vi "captureBining.vi"(0 "Image in":T1, 1 "session in":refnum<k35>, 5 "imageBinned":T1, 7 "Cam ID":u32, 9 "Binning":u32, 11 "error in (no error)":errorcluster) -> (3 "session out":refnum<k35>, 4 "Image out":T1, 15 "error out":errorcluster)   [LabVIEW 2022 SP3]
uses:
  <vilib>/vision/Image Controls.llb/IMAQ Image.ctl
  <vilib>/vision/NI_Vision_Development_Module.lvlib
panel:
  in  "Image Size":cluster{"x":i32, "y":i32}
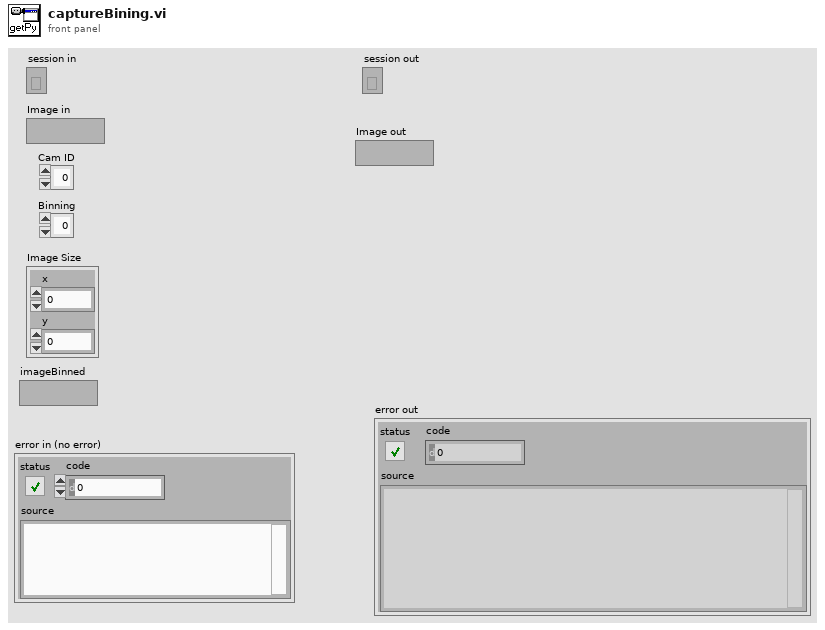
[diagram p1: front panel]
types:
  T1 = typedef "IMAQ Image.ctl" = refnum<image>
  T2 = cluster{"[0]":u32, "[1]":u32, "[2]":u32, "[3]":u32, "[4]":u32, "[5]":u32, "[6]":u32, "[7]":u32, "[8]":u32}
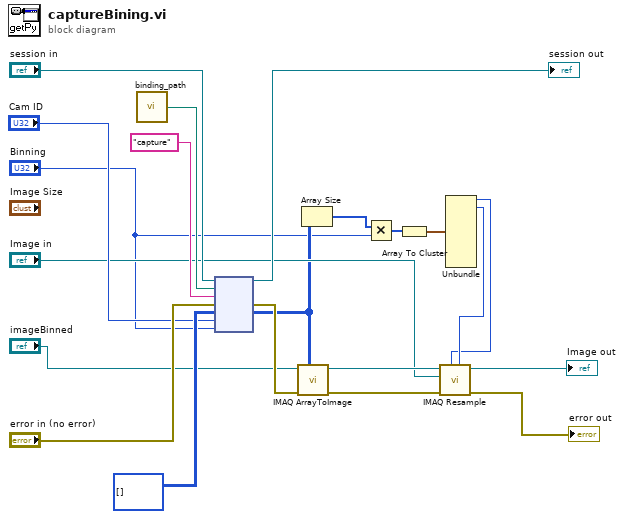
[diagram p0: block diagram]
diagram:
  n1 = call "binding_path.vi"() -> ("appended path"=w12:path)
  n2 = node("session in", w12, "capture" ("function name"), "error in (no error)", u16[][] [] ("image"), "Cam ID", "Binning") -> (→"session out":refnum<k35>, w15:errorcluster, w7:u16[][])  [unwired: 2 in, 2 out]
  n3 = call "IMAQ ArrayToImage"("Image Pixels (U16)"=w7, "error in (no error)"=w15, "Image"="imageBinned") -> ("error out"=w13:errorcluster, "Image Out"=w20:T1)  [unwired: 7 in]
  n4 = Array Size(array=w7) -> (size(s)=w6:i32[])
  n5 = Multiply(x=w6, y="Binning") -> (x*y=w4:u32[])
  n6 = Array To Cluster(array=w4) -> (cluster=w3:T2)
  n7 = Unbundle(w3) -> ("[0]"=w1:u32, "[1]"=w2:u32)  [unwired: 7 out]
  n8 = call "IMAQ Resample"("X Resolution"=w2, "Y Resolution"=w1, "error in (no error)"=w13, "Image Dst"="Image in", "Image Src"=w20) -> ("error out"=→"error out":errorcluster, "Image Dst Out"=→"Image out":T1)  [unwired: 5 in]
